vi "lm Color Enable.vi"(8 "error in (no error)":errorcluster, 10 "str_State":string, 11 "str_Color":string) -> (0 "error out":errorcluster, 2 "str_State out":string, 3 "str_Color out":string)   [LabVIEW 2018, in "LumencorDLL32.lvlib"]
doc: "This Function Enables or Disables an LE Color. Valid Colors are LE dependent. Color names should be in UPPER case (RED, GREEN etc.) The State will be either 'ON\" or \"OFF\" and in upper case.\n\n\nextern \"C\" LUMENCORDLL2B_API void lmColorEnable(char *str_Color, char *str_State);"
uses:
  LumencorDLL32.lvlib
  LumencorDLL32.dll
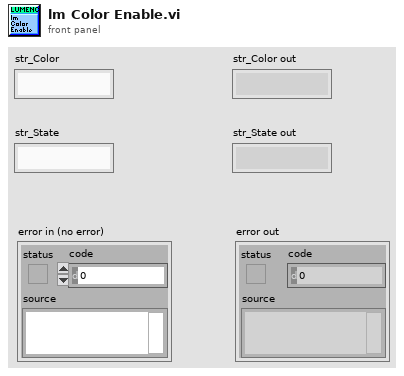
[diagram p1: front panel]
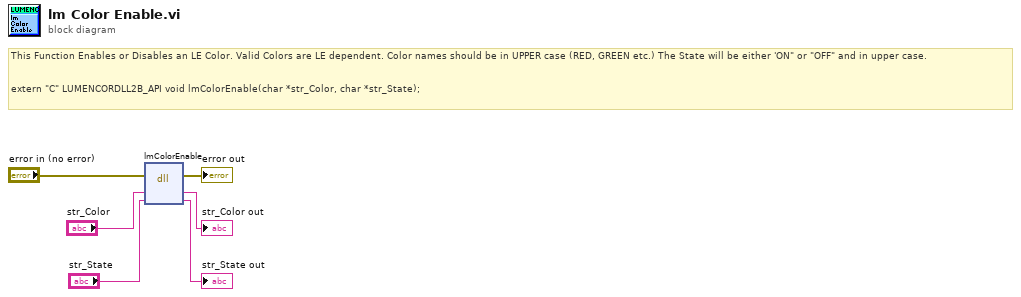
[diagram p0: block diagram]
diagram:
  # "This Function Enables or Disables an LE Color. Valid Colors are LE dependent. Color names should be in UPPER case (RED, GREEN etc.) The State will be either 'ON\" or \"OFF\" and in upper case.\n\n\nextern \"C\" LUMENCORDLL2B_API void lmColorEnable(char *str_Color, char *str_State);"
  n1 = dll-call lib="C:/Users/e14user/Documents/LabVIEW software/GitRepo/lib/SOLA/LabVIEW 2015 Library (32bit)/LumencorDLL32/LumencorDLL32.*" fn="lmColorEnable"(error in="error in (no error)", "str_Color"="str_Color", "str_State"="str_State") -> (error out=→"error out":errorcluster, "str_Color"=→"str_Color out":string, "str_State"=→"str_State out":string)  [unwired: 3 in, 1 out]
